vi "Close Tree.vi"(8 "error in (no error)":errorcluster, 11 "Connection in":refnum<class "Connection.lvclass">) -> (0 "error out":errorcluster, 3 "Connection out":refnum<class "Connection.lvclass">)   [LabVIEW 2015, in "MDSplus.lvlib" / "Connection.lvclass"]
uses:
  <vilib>/MDSplus/Classes/Connection_Class/Connection.lvclass
  <vilib>/MDSplus/Classes/Connection_Class/Connection.lvclass/Connection.ctl
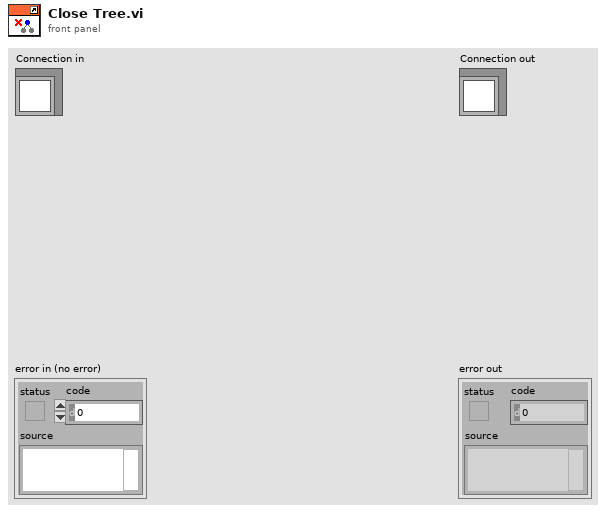
[diagram p1: front panel]
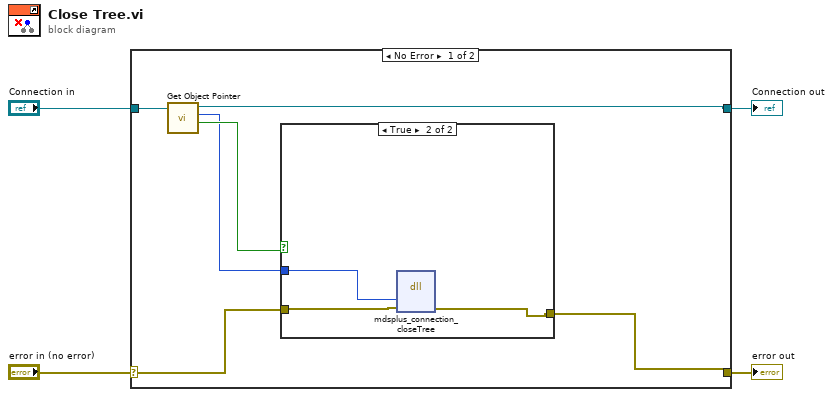
[diagram p0: block diagram]
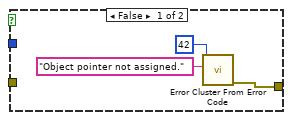
[diagram p2: hidden frame]
diagram:
  n1 = case shown="No Error" "error in (no error)" {
    selector: "error in (no error)" -> [w7 w18]
    tunnel: [w6 w18] -> w3
    tunnel: [w5 w17] -> w1
    tunnel: "Connection in" -> [w8 w17]
    frame No Error {
      n2 = call <vilib>:"Get Object Pointer.vi"("Connection in"=w8) -> ("Assigned object pointer?"=w10:bool, "Object Pointer"=w9:i64, "Connection out"=w5:refnum<class "Connection.lvclass">)  [unwired: 7 in, 1 out]
      n3 = case shown="True" w10 {
        tunnel: [w11 w15] -> w6
        tunnel: w9 -> [_ w16]
        tunnel: w7 -> [_ w14]
        frame False {
          n4 = call <vilib>:"Error Cluster From Error Code.vi"("error message (\"\")"="Object pointer not assigned." ("error message (\"\")"), "error code (0)"=42) -> ("error out"=w11:errorcluster)  [unwired: 7 in]
        }
        frame True {
          n5 = dll-call lib="MDSobjectsLVShr" fn="mdsplus_connection_closeTree"("lvConnection"=w16, w14) -> (w15:errorcluster)  [unwired: 5 in, 2 out]
        }
      }
    }
    frame Error {
    }
  }
  "error out" <- w3
  "Connection out" <- w1
